vi "State Logger Launch.vi"   [LabVIEW 2011, in "Messenging.lvlib" / "State Logger.lvclass"]
uses:
  State Logger.lvclass
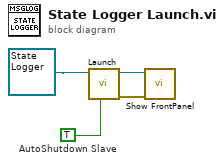
[diagram p0: block diagram]
diagram:
  w1 = TRUE  # AutoShutdown Slave
  n1 = call-dynamic "Launch.vi"("AutoShutdown Slave (F)"=w1, "Parallel Process in"=refnum<class "State Logger.lvclass"> refnum ("Parallel Process.lvlib:Messsage Logger.lvclass")) -> ("error out"=w4:errorcluster, "Parallel Process out"=w2:refnum<class "State Logger.lvclass">)  [unwired: 2 in, 6 out]
  n2 = call-dynamic "Show FrontPanel.vi"("error in (no error)"=w4, "Parallel Process in"=w2) -> ()  [unwired: 1 in, 9 out]
